vi "Buffer_Control.vi"(5 "Temp":u32[](array[numeric]), 6 "Del":cluster{"Del_Length":i32, "Del_Position":i32}, 7 "Mode":T1, 8 "error in (no error)":errorcluster caption="에러 입력(에러 없음)", 9 "Counts":u32[][](array[numeric]), 10 "Timeline":dbl[](array[numeric]) format="%#.9g", 11 "Init input":string[](array[string])) -> (0 "error out":errorcluster caption="에러 출력", 1 "Counts out":u32[][](array[numeric]), 2 "Timeline out":dbl[](array[numeric]) format="%#.9g", 3 "origin out":string[][](array[string]), 4 "Temp out":u32[](array[numeric]))   [LabVIEW 2015]
uses:
  buffer_mode.ctl
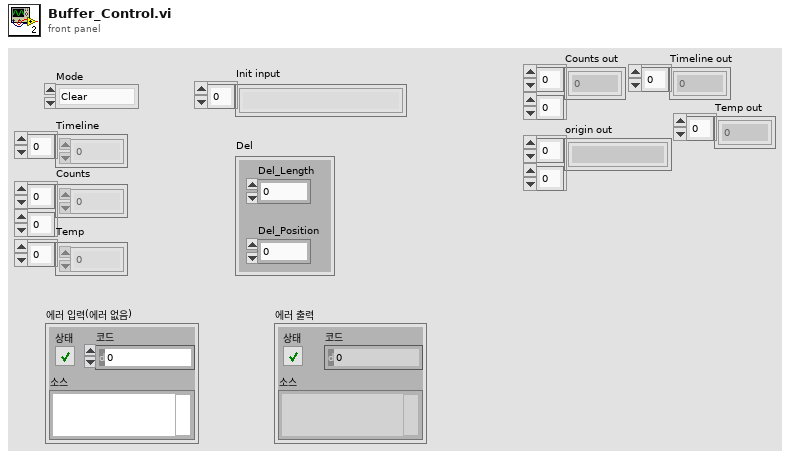
[diagram p1: front panel]
types:
  T1 = typedef "buffer_mode.ctl" = enum16{"Clear", "Init", "Add 2nd data", "Delete", "Output"}
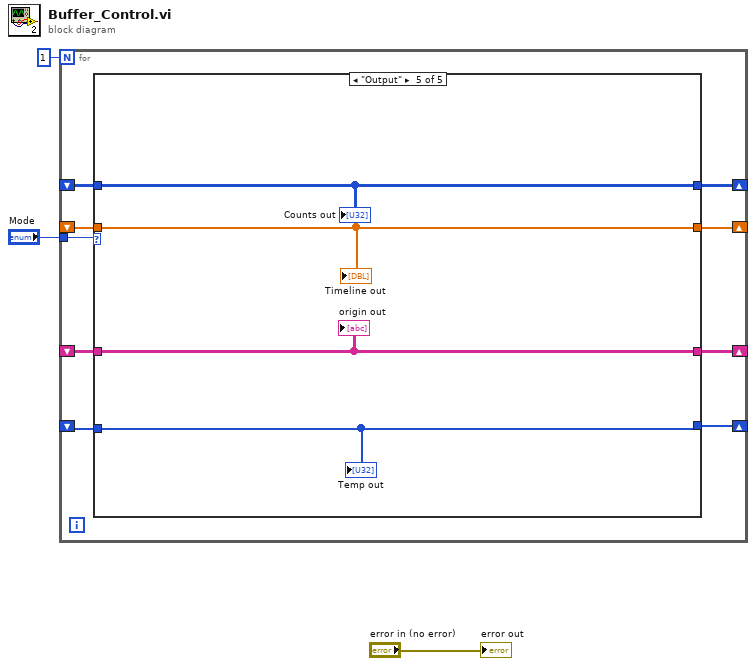
[diagram p0: block diagram]
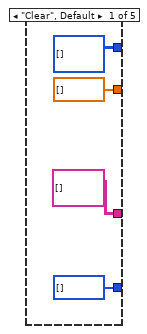
[diagram p2: hidden frame]
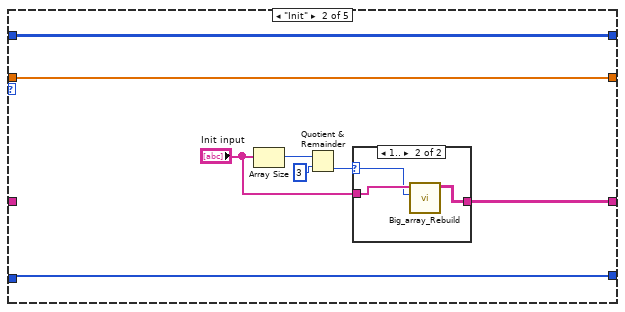
[diagram p3: hidden frame]
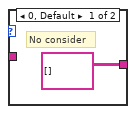
[diagram p4: hidden frame]
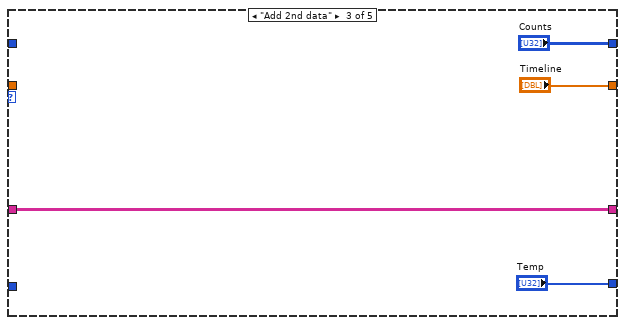
[diagram p5: hidden frame]
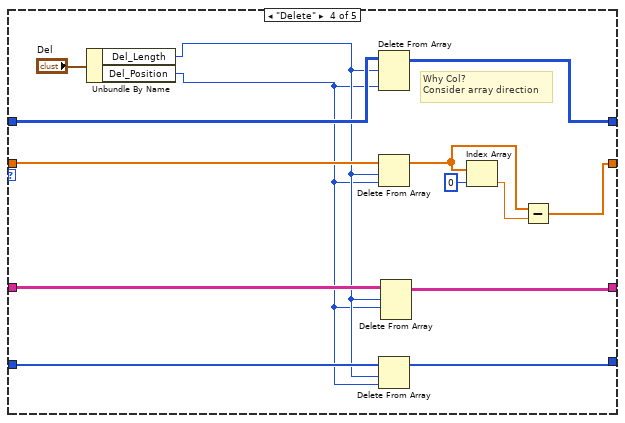
[diagram p6: hidden frame]
diagram:
  n1 = for {
    N: 1 -> [_]
    tunnel: "Mode" -> [w12]
    shift-right: [w11] -> _
    shift-left: _ -> [w10]
    shift-right: [w9] -> _
    shift-left: _ -> [w8]
    shift-right: [w7] -> _
    shift-left: _ -> [w6]
    shift-right: [w5] -> _
    shift-left: _ -> [w4]
    n2 = case shown="\"Output\"" w12 {
      tunnel: [string[][] [] w22 w32 w42 w50] -> w11
      tunnel: w10 -> [_ _ w32 w43 w50]
      tunnel: [dbl[] [] ("Timeline") w24 "Timeline" w37 w49] -> w9
      tunnel: w8 -> [_ w24 _ w44 w49]
      tunnel: [u32[][] [] ("Counts") w23 "Counts" w45 w48] -> w7
      tunnel: w6 -> [_ w23 _ w46 w48]
      tunnel: [u32[] [] ("Temp") w17 "Temp" w33 w47] -> w5
      tunnel: w4 -> [_ w17 _ w36 w47]
      frame "Clear", Default {
      }
      frame "Init" {
        n3 = Array Size(array="Init input") -> (size(s)=w21:i32)
        n4 = Quotient & Remainder(x=w21, y=3) -> (floor(x/y)=w18:i32)  [unwired: 1 out]
        n5 = case shown="1.." w18 {
          selector: w18 -> [_ w27]
          tunnel: "Init input" -> [_ w28]
          tunnel: [string[][] [] ("추가된 배열") w26] -> w22
          frame 0, Default {
            # "No consider"
          }
          frame 1.. {
            n6 = call "Big_array_Rebuild.vi"("숫자형"=w27, "Init input"=w28) -> ("추가된 배열"=w26:string[][])  [unwired: 9 in]
          }
        }
      }
      frame "Add 2nd data" {
      }
      frame "Delete" {
        # "Why Col?\nConsider array direction"
        n7 = Unbundle By Name("Del") -> ("Del_Length"=w35:i32, "Del_Position"=w34:i32)
        n8 = Delete From Array(array=w46, length=w35, index (col)=w34) -> (array with subset deleted=w45:u32[][])  [unwired: 1 in, 1 out]
        n9 = Delete From Array(array=w44, length=w35, index=w34) -> (array with subset deleted=w38:dbl[])  [unwired: 1 out]
        n10 = Delete From Array(array=w36, length=w35, index=w34) -> (array with subset deleted=w33:u32[])  [unwired: 1 out]
        n11 = Delete From Array(array=w43, length=w35, index (row)=w34) -> (array with subset deleted=w42:string[][])  [unwired: 1 in, 1 out]
        n12 = Index Array(array=w38, index=0 ("인덱스")) -> (element=w39:dbl)
        n13 = Subtract(x=w38, y=w39) -> (x-y=w37:dbl[])
      }
      frame "Output" {
        "Counts out" <- w48
        "Timeline out" <- w49
        "origin out" <- w50
        "Temp out" <- w47
      }
    }
  }
  "error out" <- "error in (no error)"
